vi "Create SimpleText.vi"(8 "error in (no error)":errorcluster, 10 "simpleText":string, 11 "ooWriter in":refnum<class "ooWriter.lvclass">) -> (0 "error out":errorcluster, 2 "SimpleText":refnum<k24>, 3 "ooWriter out":refnum<class "ooWriter.lvclass">)   [LabVIEW 2009, in "ooWriter.lvclass"]
uses:
  ooWriter.lvclass
  C:/Projets/LAVAG/OpenOfficeRGT/AODL/DLLs/AODL.dll
  ooWriter.lvclass/ooWriter.ctl
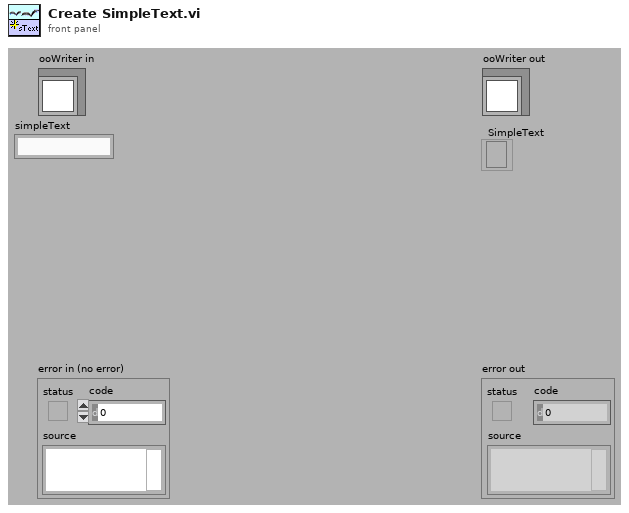
[diagram p1: front panel]
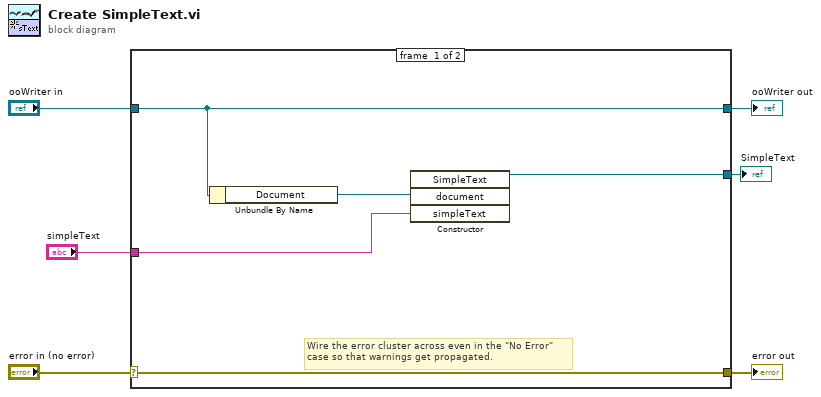
[diagram p0: block diagram]
diagram:
  n1 = case shown="No Error" "error in (no error)" {
    selector: "error in (no error)" -> [w11 w13]
    tunnel: [w11 w13] -> w5
    tunnel: [w10 w12] -> w3
    tunnel: "ooWriter in" -> [w10 w12]
    tunnel: "simpleText" -> [w8 _]
    tunnel: [w7 _] -> w1
    frame #0 {
      # "Wire the error cluster across even in the \"No Error\"\ncase so that warnings get propagated."
      n2 = Unbundle By Name(w10) -> ("Document"=w9:refnum<k24>)
      n3 = constructor class="SimpleText"("document"=w9, "simpleText"=w8) -> (reference out=w7:refnum<k24>)  [unwired: 3 in, 4 out]
    }
    frame #1 {
    }
  }
  "error out" <- w5
  "ooWriter out" <- w3
  "SimpleText" <- w1
